vi "SortLevels.vi"(11 "rule in":T1) -> (3 "rule out":T1)   [LabVIEW 2017, in "TrendAlarm.lvlib"]
uses:
  <vilib>/addons/InsightCM/Devices/Shared/Common/TrendAlarm/TrendAlarm.lvlib
  <vilib>/addons/InsightCM/MessageBus/Base/controls/TrendAlarmRule.ctl
  <vilib>/addons/InsightCM/MessageBus/Base/controls/TrendAlarmLevel.ctl
  <vilib>/addons/InsightCM/MessageBus/Base/controls/AlarmAction.ctl
  <vilib>/addons/InsightCM/MessageBus/Base/controls/KeyValuePair.ctl
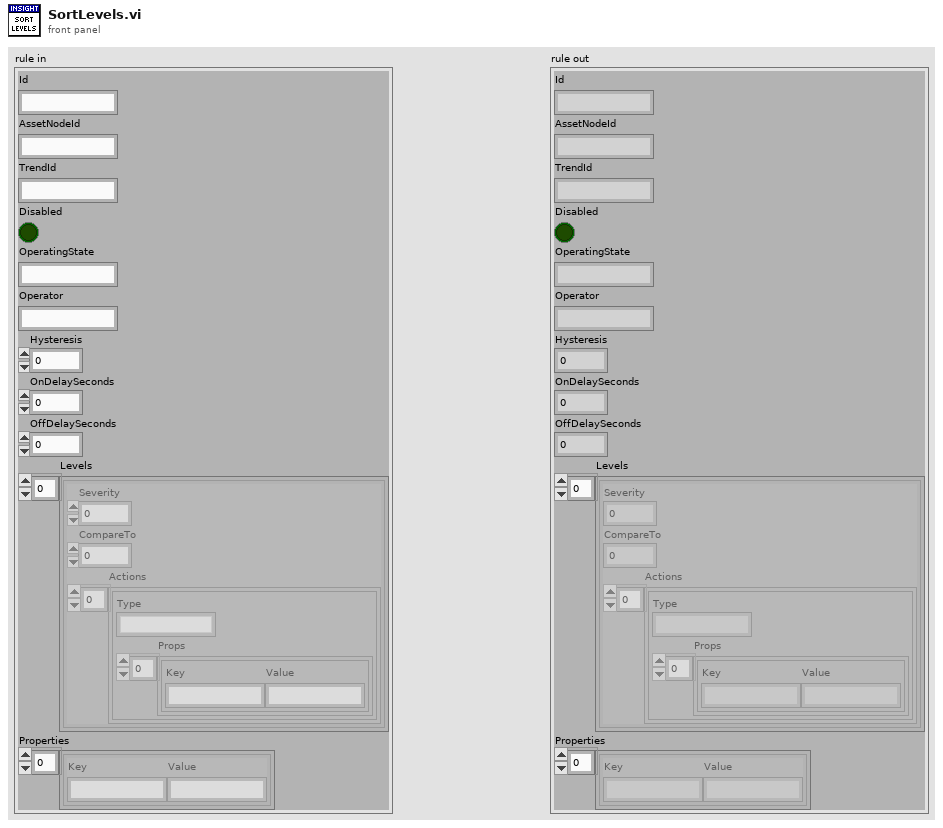
[diagram p1: front panel]
types:
  T1 = typedef "TrendAlarmRule.ctl" = cluster{"Id":string, "AssetNodeId":string, "TrendId":string, "Disabled":bool, "OperatingState":string, "Operator":string, "Hysteresis":dbl, "OnDelaySeconds":dbl, "OffDelaySeconds":dbl, "Levels":T2[], "Properties":T4[]}
  T2 = typedef "TrendAlarmLevel.ctl" = cluster{"Severity":i32, "CompareTo":dbl, "Actions":T3[]}
  T3 = typedef "AlarmAction.ctl" = cluster{"Type":string, "Props":T4[]}
  T4 = typedef "KeyValuePair.ctl" = cluster{"Key":string, "Value":string}
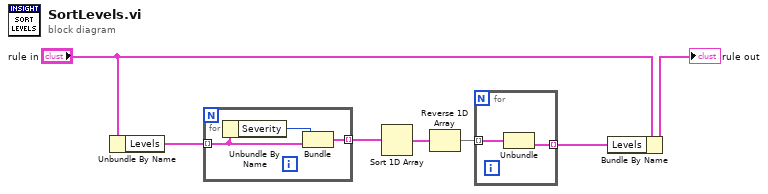
[diagram p0: block diagram]
diagram:
  n1 = Unbundle By Name("rule in") -> ("Levels"=w7:T2[])
  n2 = for {
    tunnel: w7 -> [w10] mode=indexing
    tunnel: [w8] -> w6 mode=indexing
    n3 = Unbundle By Name(w10) -> ("Severity"=w9:i32)
    n4 = Bundle("Severity"=w9, "Level"=w10) -> (w8:cluster{"Severity":i32, "Level":T2})  [unwired: 1 in]
  }
  n5 = Sort 1D Array(array=w6) -> (sorted array=w5:cluster{"Severity":i32, "Level":T2}[])
  n6 = Reverse 1D Array(array=w5) -> (reversed array=w4:cluster{"Severity":i32, "Level":T2}[])
  n7 = for {
    tunnel: w4 -> [w12] mode=indexing
    tunnel: [w11] -> w1 mode=indexing
    n8 = Unbundle(w12) -> ("Level"=w11:T2)  [unwired: 1 out]
  }
  n9 = Bundle By Name(cluster="rule in", "Levels"=w1) -> (→"rule out":T1)
